vi "ElevLimits.vi"(7 "PowerIn":dbl) -> (2 "BotLimit":bool, 3 "PowerOut":dbl)   [LabVIEW 2017]
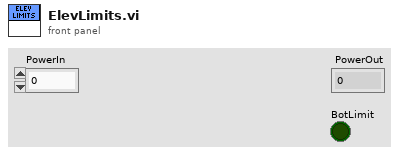
[diagram p1: front panel]
types:
  T1 = typedef "WPI_SwitchDevRef.ctl" = cluster{"DevStatus":errorcluster, "DIO Channel":T2, "CntIndex":T3, "Normally Closed":bool}
  T2 = typedef "FPGA_DIOChannel.ctl" = enum8{"DIO 0", "DIO 1", "DIO 2", "DIO 3", "DIO 4", "DIO 5", "DIO 6", "DIO 7", "DIO 8", "DIO 9", "DIO MXP 0", "DIO MXP 1", "DIO MXP 2", "DIO MXP 3", "DIO MXP 4", "DIO MXP 5", "DIO MXP 6", "DIO MXP 7", "DIO MXP 8", "DIO MXP 9", "DIO MXP 10", "DIO MXP 11", "DIO MXP 12", "DIO MXP 13", "DIO MXP 14", "DIO MXP 15", "SPI Port CS1", "SPI Port CS2", "SPI Port CS3", "SPI Port MISO", "SPI Port MOSI", "Invalid"}
  T3 = typedef "FPGA_CounterCtrSystemIndex.ctl" = enum8{"Ctr 0", "Ctr 1", "Ctr 2", "Ctr 3", "Ctr 4", "Ctr 5", "Ctr 6", "Ctr 7", "Invalid"}
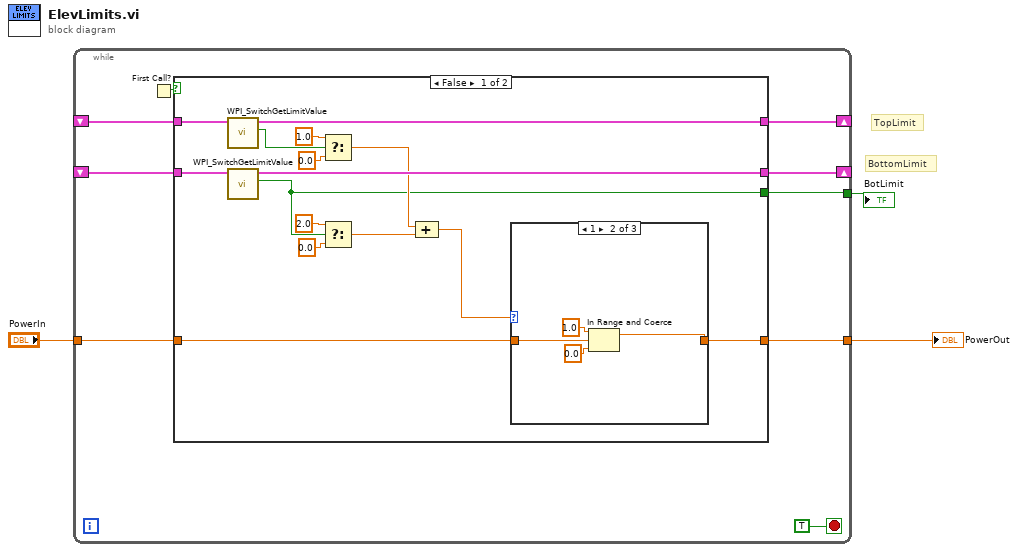
[diagram p0: block diagram]
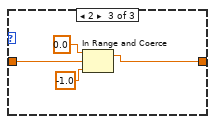
[diagram p3: hidden frame]
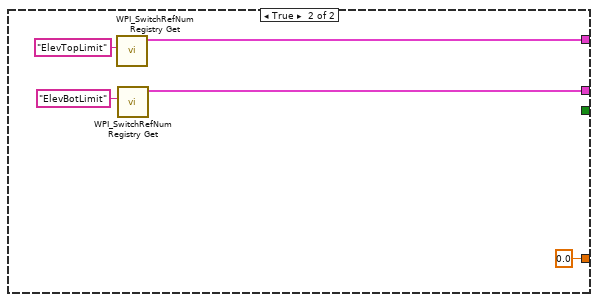
[diagram p4: hidden frame]
diagram:
  # "BottomLimit"
  # "TopLimit"
  n1 = while {
    shift-right: [w9] -> _
    shift-left: _ -> [w7]
    shift-right: [w10] -> _
    shift-left: _ -> [w8]
    tunnel: "PowerIn" -> [w6]
    tunnel: [w5] -> w2
    tunnel: [w4] -> w1
    stop <- TRUE stop-if-true
    n2 = First Call?() -> (First Call?: T/F=w11:bool)
    n3 = case shown="False" w11 {
      tunnel: [w24 w39] -> w10
      tunnel: [w26 w38] -> w9
      tunnel: w8 -> [w25 _]
      tunnel: w7 -> [w27 _]
      tunnel: w6 -> [w15 _]
      tunnel: [w14 0.0 ("upper limit")] -> w5
      tunnel: [w13 _] -> w4
      frame False {
        n4 = call <vilib>:"WPI_SwitchGetLimitValue.vi"("SwitchDevRef"=w27) -> ("Switch Pressed"=w22:bool, "SwitchDevRef"=w26:T1)  [unwired: 8 in, 1 out]
        n5 = call <vilib>:"WPI_SwitchGetLimitValue.vi"("SwitchDevRef"=w25) -> ("Switch Pressed"=w13:bool, "SwitchDevRef"=w24:T1)  [unwired: 8 in, 1 out]
        n6 = Select(t=1.0, s=w22, f=0.0) -> (s? t:f=w19:dbl)
        n7 = Select(t=2.0, s=w13, f=0.0) -> (s? t:f=w16:dbl)
        n8 = Compound Arithmetic op=ADD(w19, w16) -> (w23:dbl)
        n9 = case shown="1" w23 {
          tunnel: w15 -> [w28 w32 w36]
          tunnel: [w28 w31 w33] -> w14
          frame 0, Default {
          }
          frame 1 {
            n10 = In Range and Coerce(upper limit=1.0, x=w32, lower limit=0.0) -> (coerced(x)=w31:dbl)  [unwired: 1 out]
          }
          frame 2 {
            n11 = In Range and Coerce(upper limit=0.0, x=w36, lower limit=-1.0) -> (coerced(x)=w33:dbl)  [unwired: 1 out]
          }
        }
      }
      frame True {
        n12 = call <vilib>:"WPI_SwitchRefNum Registry Get.vi"("refnum name"="ElevTopLimit") -> ("SwitchDevRef"=w38:T1)  [unwired: 9 in, 1 out]
        n13 = call <vilib>:"WPI_SwitchRefNum Registry Get.vi"("refnum name"="ElevBotLimit") -> ("SwitchDevRef"=w39:T1)  [unwired: 9 in, 1 out]
      }
    }
  }
  "PowerOut" <- w2
  "BotLimit" <- w1
